vi "toggleONsubvi.vi"() -> ()   [LabVIEW 2017]
uses:
  <vilib>/ULx/Create Channel.llb/ULx Create Channel (DO-Digital Output).vi
  <vilib>/ULx/Write.llb/ULx Write (Digital Bool 1Line 1Point).vi
panel:
  out "error out":errorcluster
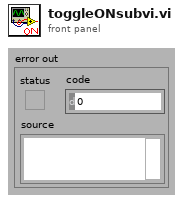
[diagram p1: front panel]
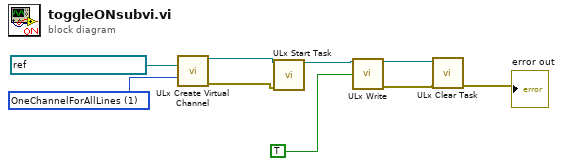
[diagram p0: block diagram]
diagram:
  w8 = 1 items=["OneChannelForEachLine", "OneChannelForAllLines"] ("line grouping")
  n1 = call-poly <vilib>:"ULx Create Virtual Channel.vi"("lines"=refnum<k21> "Dev0/1stPortCL/Do0", "line grouping"=w8) -> ("task out"=w7:refnum<k24>, "error out"=w6:errorcluster)  [unwired: 12 in]
  n2 = call <vilib>:"ULx Start Task.vi"("task in"=w7, "error in"=w6) -> ("task out"=w5:refnum<k24>)  [unwired: 12 in, 1 out]
  n3 = call-poly <vilib>:"ULx Write.vi"("task in"=w5, "data"=TRUE) -> ("task out"=w3:refnum<k24>, "error out"=w2:errorcluster)  [unwired: 11 in, 1 out]
  n4 = call <vilib>:"ULx Clear Task.vi"("task in"=w3, "error in"=w2) -> ("error out"=→"error out":errorcluster)  [unwired: 13 in]
